vi "声音录音次vi.vi"() -> ()   [LabVIEW 2024]
uses:
  <vilib>/sound2/lvsound2.llb/Sampling Mode.ctl
  <vilib>/sound2/lvsound2.llb/Sound Data Format.ctl
  <vilib>/sound2/lvsound2.llb/Sound File Write Open.vi
  <vilib>/sound2/lvsound2.llb/Sound Input Read (DBL).vi
  <vilib>/express/express analysis/Spectral/Block/exnSpectralBlock spectral measurements RMS poly.vi
  <vilib>/express/express analysis/Spectral/Block/exnSpectralBlock spectral measurements RMS array WFM.vi
  <vilib>/sound2/lvsound2.llb/Sound File Write (DBL).vi
  <vilib>/sound2/lvsound2.llb/Sound File Info (path).vi
  <vilib>/sound2/lvsound2.llb/Sound File Read Open.vi
  <vilib>/sound2/lvsound2.llb/Sound File Read (DBL).vi
  <vilib>/sound2/lvsound2.llb/Sound Output Write (DBL).vi
  <vilib>/express/express analysis/Spectral/XNode/ExpressSpectralMeasurementsBlockNode.xnode
panel:
  in  "device ID 2":u32 caption="设备ID"
  in  "number of samples/ch 2":i32=100000 caption="每通道采样数"
  in  "播放声音":bool
  in  "停止":bool
  in  "开始录音":bool
  in  "?":enum32{"选项卡 1", "选项卡 2"}(tab)
  out "波形图":waveform(dbl)[](graph)
  out "波形图 2":cluster{"f0":dbl, "df":dbl, "magnitude":dbl[]}[](graph)
  out "error out":errorcluster caption="错误输出"
  in  "device ID":u32 caption="设备ID"
  in  "sound format":T1={"sample rate (S/s)"=22050.0, "number of channels"=2, "bits per sample"=16} caption="声音格式"
  in  "sample mode":T2=1 caption="采样模式" items=["有限采样", "连续采样"]
  in  "number of samples/ch":i32=100000 caption="每通道采样数"
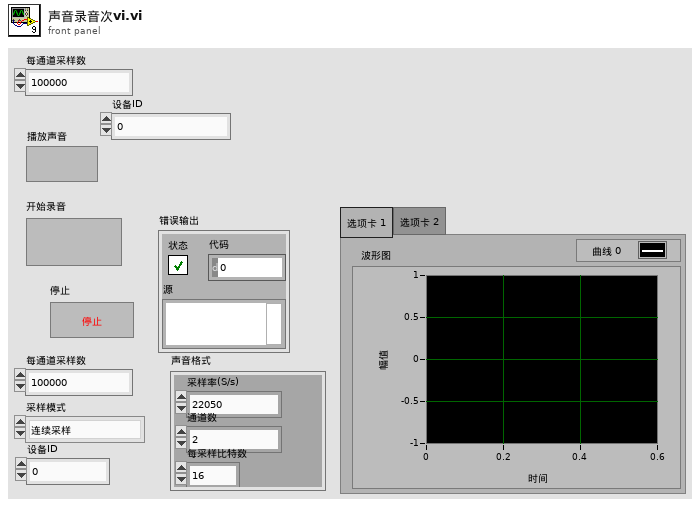
[diagram p1: front panel]
types:
  T1 = typedef "Sound Data Format.ctl" = cluster{"sample rate (S/s)":dbl, "number of channels":i32, "bits per sample":i32}
  T2 = typedef "Sampling Mode.ctl" = i32
  T3 = cluster{"averaging mode":u16, "weighting mode":u16, "number of averages":u32}
  T4 = cluster{"dB On (F)":bool, "unwrap phase (F)":bool, "convert to degree (F)":bool}
  T5 = typedef "Sound Input Task ID.ctl" = u32
  T6 = typedef "Sound File Refnum.ctl" = refnum<file>
  T7 = typedef "Sound Output Task ID.ctl" = u32
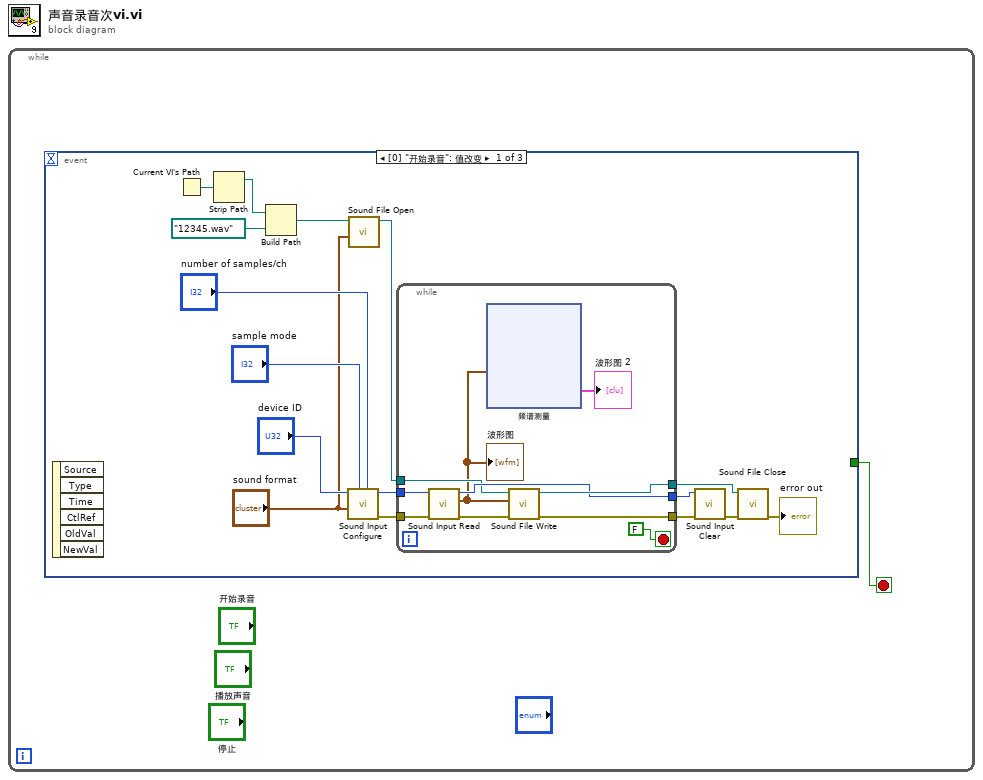
[diagram p0: block diagram]
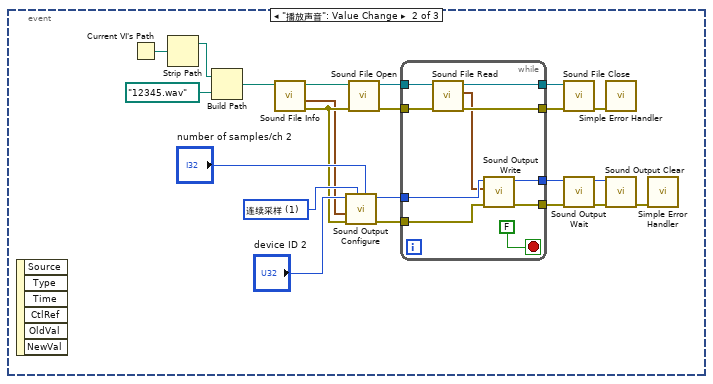
[diagram p2: hidden frame]
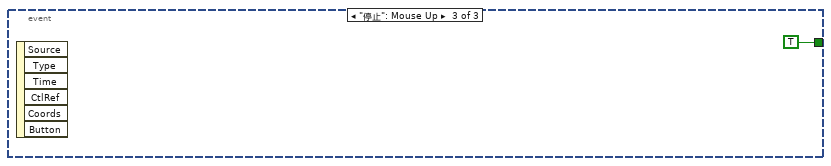
[diagram p3: hidden frame]
diagram:
  n1 = while {
    stop <- w1 stop-if-true
    n2 = event shown="[0] \"开始录音\": 值改变" {
      selector: _ -> [_ _ _]
      dyn-events: _ -> [_ _ _]
      timeout: _ -> [_ _ _]
      tunnel: [_ _ TRUE] -> w1
      event "开始录音": Value Change {
        n3 = event-data() -> ()  [unwired: 1 in, 6 out]
        n4 = Current VI's Path() -> (path=w8:path)
        n5 = Strip Path(path=w8) -> (stripped path=w7:path)  [unwired: 1 out]
        n6 = Build Path(base path=w7, name or relative path=path "12345.wav" ("名称或相对路径")) -> (appended path=w6:path)
        n7 = call <vilib>:"Sound Input Configure.vi"("number of samples/ch"="number of samples/ch", "sample mode"="sample mode", "sound format"="sound format", "device ID"="device ID") -> ("error out"=w14:errorcluster, "task ID"=w10:T5)  [unwired: 6 in]
        n8 = call-poly <vilib>:"Sound File Open.vi"("sound format"="sound format", "path"=w6) -> ("sound file refnum"=w5:T6)  [unwired: 8 in, 1 out]
        n9 = while {
          tunnel: [w24] -> w11
          tunnel: w5 -> [w21]
          tunnel: w14 -> [w27]
          tunnel: [w25] -> w13
          tunnel: w10 -> [w23]
          tunnel: [w22] -> w9
          stop <- FALSE stop-if-true
          n10 = call-poly <vilib>:"Sound Input Read.vi"("error in (no error)"=w27, "task ID"=w23) -> ("error out"=w26:errorcluster, "data"=w20:waveform(dbl)[], "task ID out"=w22:T5)  [unwired: 7 in]
          "波形图" <- w20
          n11 = xnode "频谱测量"("信号"=w20) -> ("测量输出"=→"波形图 2":cluster{"f0":dbl, "df":dbl, "magnitude":dbl[]}[])  [unwired: 1 in, 2 out]
          n12 = call-poly <vilib>:"Sound File Write.vi"("error in (no error)"=w26, "data"=w20, "sound file refnum"=w21) -> ("error out"=w25:errorcluster, "sound file refnum out"=w24:T6)  [unwired: 7 in]
        }
        n13 = call <vilib>:"Sound Input Clear.vi"("error in (no error)"=w13, "task ID"=w9) -> ("error out"=w12:errorcluster)  [unwired: 9 in]
        n14 = call <vilib>:"Sound File Close.vi"("error in (no error)"=w12, "sound file refnum"=w11) -> ("error out"=→"error out":errorcluster)  [unwired: 9 in]
      }
      event "播放声音": Value Change {
        w48 = T2 1 items=["有限采样", "连续采样"] ("sample mode")
        n15 = event-data() -> ()  [unwired: 1 in, 6 out]
        n16 = Current VI's Path() -> (path=w59:path)
        n17 = Strip Path(path=w59) -> (stripped path=w58:path)  [unwired: 1 out]
        n18 = Build Path(base path=w58, name or relative path=path "12345.wav" ("名称或相对路径")) -> (appended path=w56:path)
        n19 = call-poly <vilib>:"Sound File Info.vi"("path"=w56) -> ("error out"=w47:errorcluster, "sound format"=w38:T1, "path out"=w53:path)  [unwired: 7 in, 1 out]
        n20 = call <vilib>:"Sound Output Configure.vi"("number of samples/ch"="number of samples/ch 2", "sample mode"=w48, "error in (no error)"=w47, "sound format"=w38, "device ID"="device ID 2") -> ("error out"=w46:errorcluster, "task ID"=w41:T7)  [unwired: 5 in]
        n21 = call-poly <vilib>:"Sound File Open.vi"("error in (no error)"=w47, "path"=w53) -> ("error out"=w55:errorcluster, "sound file refnum"=w52:T6)  [unwired: 8 in]
        n22 = while {
          tunnel: w55 -> [w69]
          tunnel: [w68] -> w54
          tunnel: w52 -> [w67]
          tunnel: [w66] -> w51
          tunnel: w46 -> [w65]
          tunnel: [w64] -> w45
          tunnel: w41 -> [w62]
          tunnel: [w61] -> w40
          stop <- FALSE stop-if-true
          n23 = call-poly <vilib>:"Sound File Read.vi"("error in (no error)"=w69, "sound file refnum"=w67) -> ("error out"=w68:errorcluster, "data"=w60:waveform(dbl)[], "sound file refnum out"=w66:T6)  [unwired: 5 in, 2 out]
          n24 = call-poly <vilib>:"Sound Output Write.vi"("error in (no error)"=w65, "data"=w60, "task ID"=w62) -> ("error out"=w64:errorcluster, "task ID out"=w61:T7)  [unwired: 7 in]
        }
        n25 = call <vilib>:"Sound File Close.vi"("error in (no error)"=w54, "sound file refnum"=w51) -> ("error out"=w43:errorcluster)  [unwired: 9 in]
        n26 = call <vilib>:"Sound Output Wait.vi"("error in (no error)"=w45, "task ID"=w40) -> ("error out"=w44:errorcluster, "task ID out"=w39:T7)  [unwired: 8 in]
        n27 = call <vilib>:"Simple Error Handler.vi"("error in (no error)"=w43) -> ()  [unwired: 4 in, 5 out]
        n28 = call <vilib>:"Sound Output Clear.vi"("error in (no error)"=w44, "task ID"=w39) -> ("error out"=w42:errorcluster)  [unwired: 9 in]
        n29 = call <vilib>:"Simple Error Handler.vi"("error in (no error)"=w42) -> ()  [unwired: 4 in, 5 out]
      }
      event "停止": Mouse Up {
        n30 = event-data() -> ()  [unwired: 1 in, 6 out]
      }
    }
  }
